vi "GOMDBTS2048 is Multi Measurement.vi"(8 "error in (no error)":errorcluster, 10 "calibration":i32, 11 "handle":i32) -> (0 "error out":errorcluster, 2 "function return":i32, 3 "value":bool)   [LabVIEW 2015, in "GOMDBTS2048.lvlib"]
doc: "GOBTS2048DLL int __stdcall GOMDBTS2048_isMultiMeasurement(int handle, int calibration, bool* value);"
uses:
  GOMDBTS2048.lvlib
  runtime/GOMDBTS2048.dll
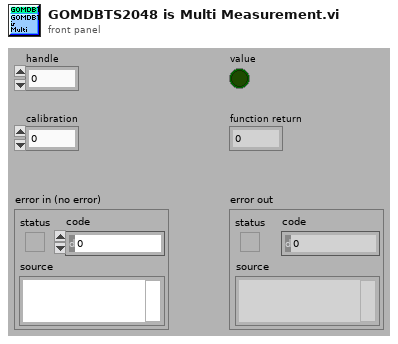
[diagram p1: front panel]
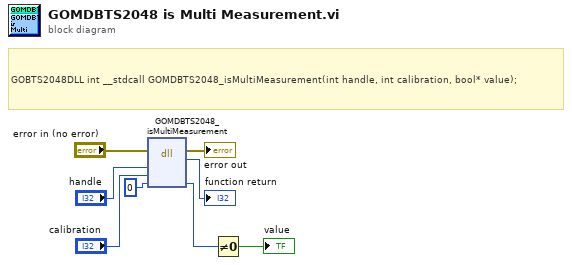
[diagram p0: block diagram]
diagram:
  # "GOBTS2048DLL int __stdcall GOMDBTS2048_isMultiMeasurement(int handle, int calibration, bool* value);"
  n1 = dll-call lib="C:/Users/rkoch/Documents/GO_Library/runtime/GOMDBTS2048.*" fn="GOMDBTS2048_isMultiMeasurement"(error in="error in (no error)", "handle"="handle", "calibration"="calibration", "value"=u8 0) -> (error out=→"error out":errorcluster, →"function return":i32, "value"=w3:u8)  [unwired: 4 in, 1 out]
  n2 = Not Equal To 0?(x=w3) -> (x != 0?=→"value":bool)
